vi "SshOpen.vi"(2 "pattern":string, 3 "host":string, 4 "username":string, 8 "password":string, 9 "error in (no error)":errorcluster) -> (0 "SshStream":refnum<k24>, 6 "error out":errorcluster, 7 "Login Answer":string)   [LabVIEW 2009]
uses:
  C:/Ohana/LV2009/OhanaOS-LV81/Instruments/Keyword/Controller/Tamir.sharpSsh.dll
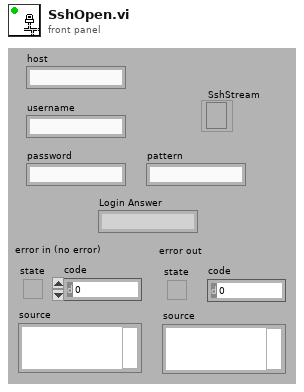
[diagram p1: front panel]
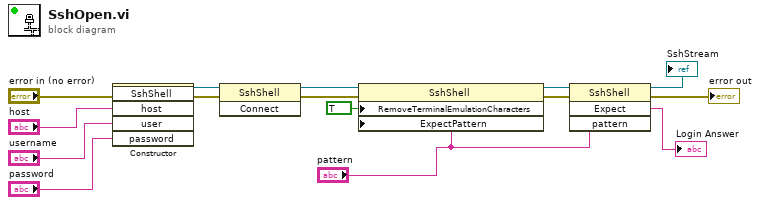
[diagram p0: block diagram]
diagram:
  n1 = constructor class="SshShell"(error in="error in (no error)", "host"="host", "user"="username", "password"="password") -> (reference out=w4:refnum<k24>, error out=w5:errorcluster)  [unwired: 2 in, 4 out]
  n2 = invoke class="SshShell" method="Connect"(reference=w4, error in=w5) -> (reference out=w2:refnum<k24>, error out=w3:errorcluster)  [unwired: 1 in, 1 out]
  n3 = property class="SshShell"(reference=w2, error in=w3, "RemoveTerminalEmulationCharacters"=TRUE, "ExpectPattern"="pattern") -> (reference out=w8:refnum<k24>, error out=w9:errorcluster)
  n4 = invoke class="SshShell" method="Expect"(reference=w8, error in=w9, "pattern"="pattern") -> (reference out=→"SshStream":refnum<k24>, error out=→"error out":errorcluster, "Expect"=→"Login Answer":string)  [unwired: 1 in, 1 out]
